vi "Suspend.vi"(8 "error in (no error)":errorcluster, 9 "Old data":T1={"Channels to measure"=[1.0], "Record heater"=FALSE, "Set point"=0.0, "Set Heater Range"=enum."Off", "Control"=FALSE, "Approach"=enum."Instant", "Ramp rate, K/min"=1.0, "Control Channel"=1, "P"=0.0, "I"=0.0, "D"=0.0, "Suspend heater"=FALSE}, 10 "New data":T1={"Channels to measure"=[1.0], "Record heater"=FALSE, "Set point"=0.0, "Set Heater Range"=enum."Off", "Control"=FALSE, "Approach"=enum."Instant", "Ramp rate, K/min"=1.0, "Control Channel"=1, "P"=0.0, "I"=0.0, "D"=0.0, "Suspend heater"=FALSE}, 11 "Neocera LTC-21 in":refnum<class "Neocera LTC-21.lvclass">) -> (0 "error out":errorcluster, 3 "Neocera LTC-21 out":refnum<class "Neocera LTC-21.lvclass">)   [LabVIEW 2015, in "Neocera LTC-21.lvclass"]
uses:
  Neocera LTC-21.lvclass
  Neocera Front Panel Data.ctl
  Neocera Heater Ranges.ctl
  Neocera Set Point Aproach.ctl
  Neocera LTC-21.lvclass/Neocera LTC-21.ctl
  Instrument/Read VISA Resource.vi
  Instrument/Write VISA Resource.vi
panel:
  # "Temperature Monitor"
  # "Temperature Control"
  # "Temperature Monitor"
  # "Temperature Control"
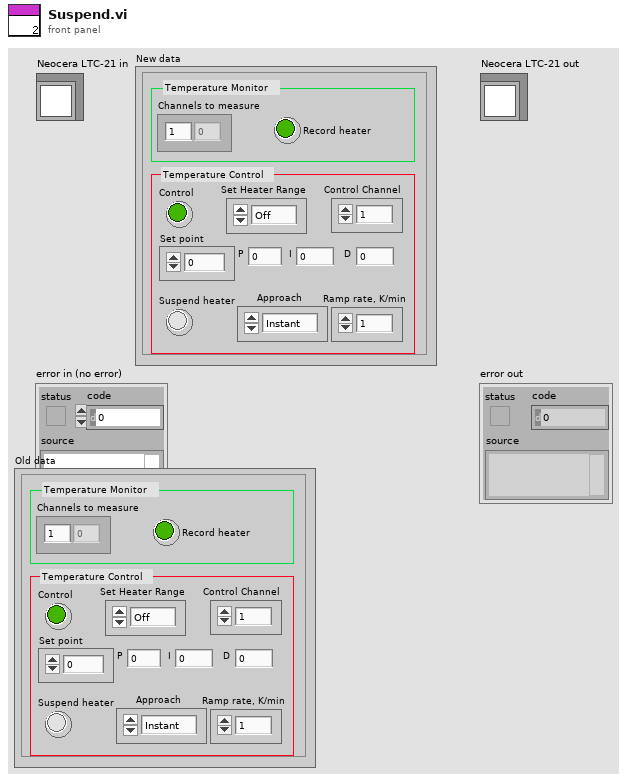
[diagram p1: front panel]
types:
  T1 = typedef "Neocera Front Panel Data.ctl" = cluster{"Channels to measure":dbl[], "Record heater":bool, "Set point":dbl, "Set Heater Range":T2, "Control":bool, "Approach":T3, "Ramp rate, K/min":dbl, "Control Channel":i16, "P":dbl, "I":dbl, "D":dbl, "Suspend heater":bool}
  T2 = typedef "Neocera Heater Ranges.ctl" = enum16{"Off", "0.05W", "0.5W", "5W", "50W"}
  T3 = typedef "Neocera Set Point Aproach.ctl" = enum16{"Instant", "Ramp"}
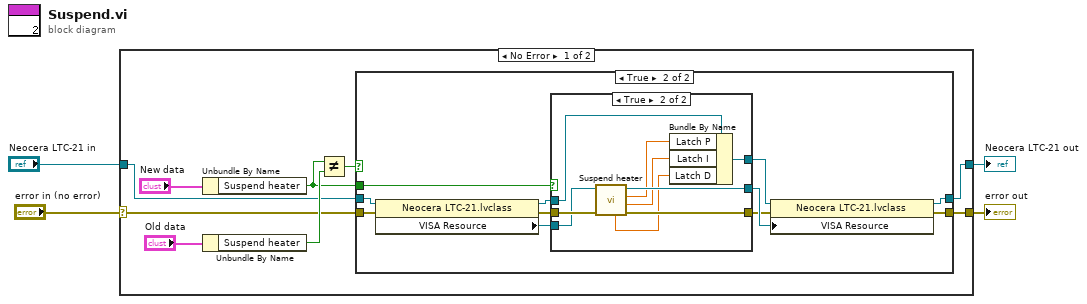
[diagram p0: block diagram]
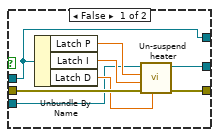
[diagram p3: hidden frame]
diagram:
  n1 = case shown="No Error" "error in (no error)" {
    selector: "error in (no error)" -> [w5 w45]
    tunnel: [w8 w45] -> w3
    tunnel: [w6 w44] -> w1
    tunnel: "Neocera LTC-21 in" -> [w7 w44]
    frame No Error {
      n2 = Unbundle By Name("New data") -> ("Suspend heater"=w9:bool)
      n3 = Unbundle By Name("Old data") -> ("Suspend heater"=w11:bool)
      n4 = Not Equal?(x=w9, y=w11) -> (x != y?=w10:bool)
      n5 = case shown="True" w10 {
        tunnel: w5 -> [w15 w19]
        tunnel: [w15 w16] -> w8
        tunnel: w9 -> [_ w26]
        tunnel: w7 -> [w14 w23]
        tunnel: [w14 w22] -> w6
        frame False {
        }
        frame True {
          n6 = property class="Neocera LTC-21.lvclass"(reference=w23, error in=w19) -> (reference out=w24:refnum<class "Neocera LTC-21.lvclass">, error out=w18:errorcluster, "VISA Resource"=w20:refnum<visa-resource-name>)
          n7 = case shown="True" w26 {
            tunnel: [w34 w43] -> w21
            tunnel: w18 -> [w33 w42]
            tunnel: [w32 w41] -> w17
            tunnel: w24 -> [w28 w40]
            tunnel: [w28 w36] -> w25
            tunnel: w20 -> [w27 w35]
            frame False {
              n8 = Unbundle By Name(w28) -> ("Latch P"=w31:dbl, "Latch I"=w30:dbl, "Latch D"=w29:dbl)
              n9 = call "Un-suspend heater.vi"("D"=w29, "error in (no error)"=w33, "I"=w30, "P"=w31, "VISA Refnum in"=w27) -> ("error out"=w32:errorcluster, "VISA Refnum out"=w34:refnum<visa-resource-name>)  [unwired: 5 in]
            }
            frame True {
              n10 = call "Suspend heater.vi"("error in (no error)"=w42, "VISA resource name"=w35) -> ("error out"=w41:errorcluster, "I"=w38:dbl, "P"=w39:dbl, "VISA resource name out"=w43:refnum<visa-resource-name>, "D"=w37:dbl)  [unwired: 4 in, 1 out]
              n11 = Bundle By Name(cluster=w40, "Latch P"=w39, "Latch I"=w38, "Latch D"=w37) -> (w36:refnum<class "Neocera LTC-21.lvclass">)
            }
          }
          n12 = property class="Neocera LTC-21.lvclass"(reference=w25, error in=w17, "VISA Resource"=w21) -> (reference out=w22:refnum<class "Neocera LTC-21.lvclass">, error out=w16:errorcluster)
        }
      }
    }
    frame Error {
    }
  }
  "error out" <- w3
  "Neocera LTC-21 out" <- w1
